vi "Simulated Acquisition Template (Host).vi"() -> ()   [LabVIEW 2016]
uses:
  <vilib>/FPGAPlugInAG/roboRIO/niLvFpga_Open_roboRIO.vi
  <vilib>/rvi/interface/common/dynamic/niFpgaDynamicAddResources.vi
  <vilib>/FPGAPlugInAG/Dynamic/niLvFpga_Download_Dynamic.vi
  <vilib>/FPGAPlugInAG/Dynamic/niLvFpga_Run_Dynamic.vi
  <vilib>/visionFPGA/Basics/Configure Image Transfer to Target/IMAQ FPGA Configure Image Transfer to Target U32.vi
  <vilib>/visionFPGA/Basics/Image Transfer to Target/IMAQ FPGA Image Transfer to Target U32.vi
  <vilib>/visionFPGA/Basics/Configure Image Transfer from Target/IMAQ FPGA Configure Image Transfer from Target U8.vi
  <vilib>/Utility/error.llb/Error Cluster From Error Code.vi
  <vilib>/rvi/errors/niLvFpgaAdjustHostInterfaceError.vi
  <vilib>/visionFPGA/Basics/Image Transfer from Target/IMAQ FPGA Image Transfer from Target U8.vi
  <vilib>/FPGAPlugInAG/Dynamic/niLvFpga_Close_Dynamic.vi
  <vilib>/rvi/interface/nirviOpenFPGA/nirviOpenFPGA.xnode
  FPGA Bitfiles/ImageProcessingw_FPGATarget2_ImageProcessingw_ZcF2hsHpmf8.lvbitx
  Image Processing with Vision Assistant (FPGA).vi
  <vilib>/rvi/interface/nirviMethod/nirviMethod.xnode
  <vilib>/rvi/interface/nirviReadWriteControl/nirviReadWriteControl.xnode
  <vilib>/rvi/interface/nirviCloseFPGA/nirviCloseFPGA.xnode
  <vilib>/visionFPGA/NI_VDM_FPGA_Basics.lvlib
  NiFpgaLv.dll
  <vilib>/rvi/interface/Simulation/niFpgaSimulationCallBeginRW.vi
panel:
  out "Image 2":T1(plugin-control)
  in  "Image Folder":path=path "/VISION/Images"
  out "Error Out":errorcluster
  out "Image":T1(plugin-control)
  in  "Stop":bool
  # "Overview: Demonstrates how to cycle through a folder of images, transfer the images to a FPGA target for processing, and retrieve the processed images for display or further processing on the host.\nRequirements:\n- LabVIEW FPGA\n- Vision Development Module\nInstructions:\n1. Select the folder containing the images to use.  For a Real-Time target it may be necessary to copy the images to the target first.\n2. Run the VI."
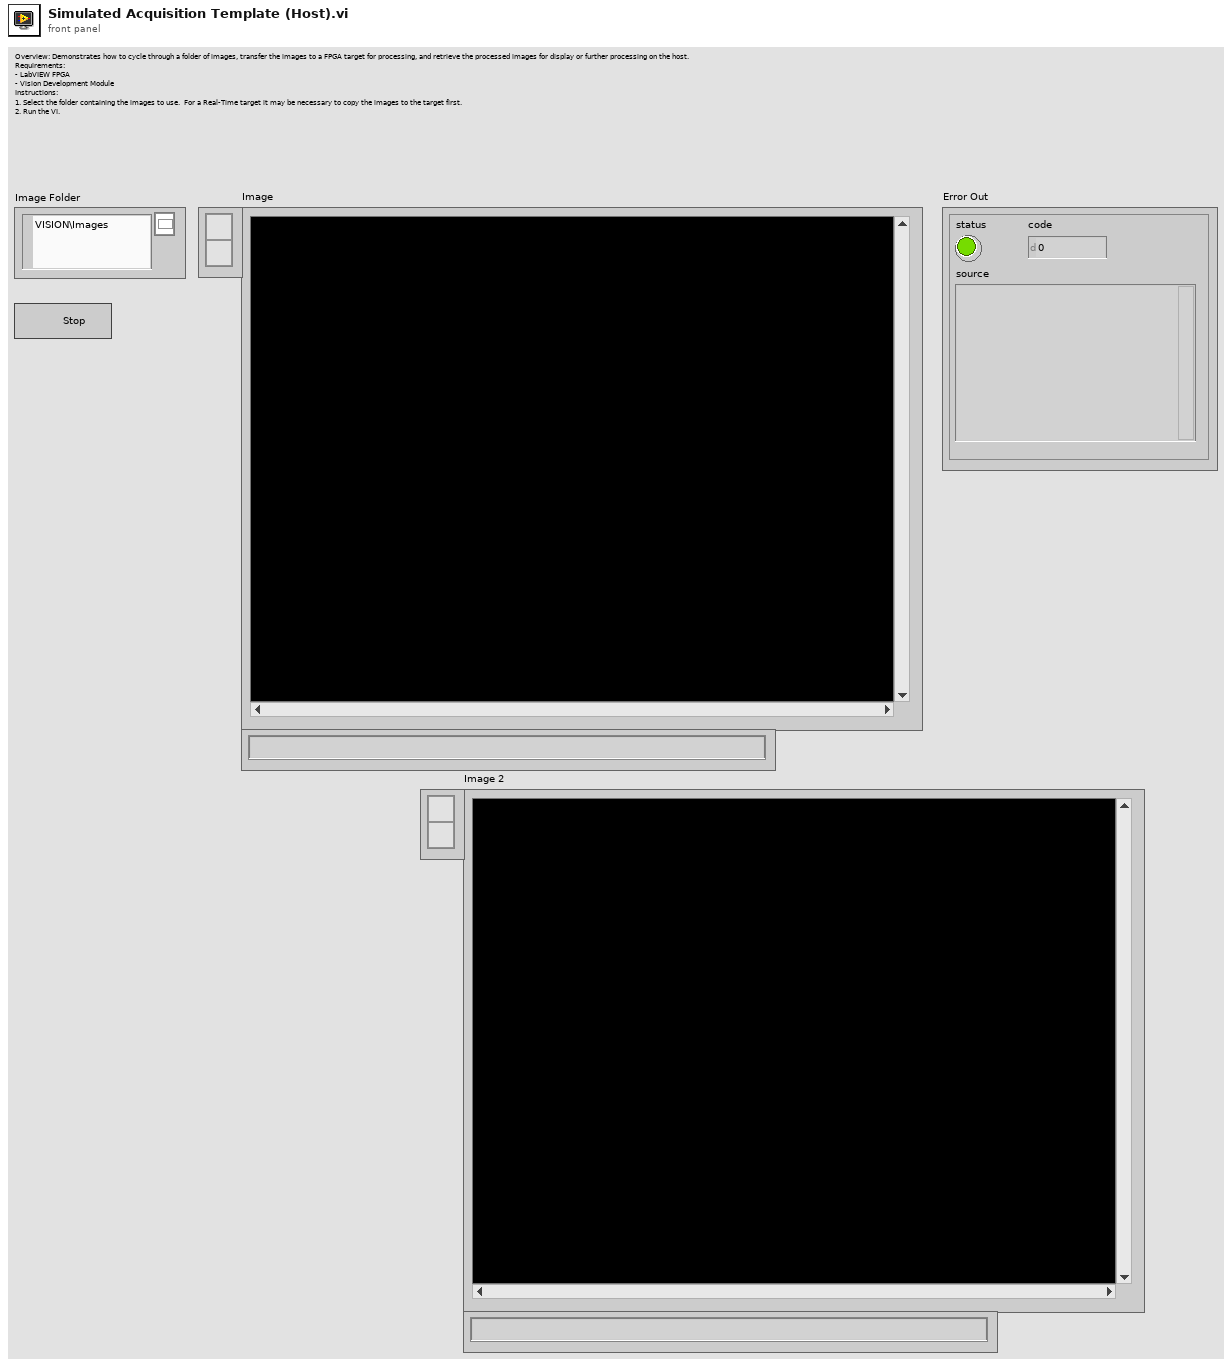
[diagram p1: front panel]
types:
  T1 = typedef "IMAQ Image.ctl" = refnum<image>
  T2 = typedef "Image Type" = u32
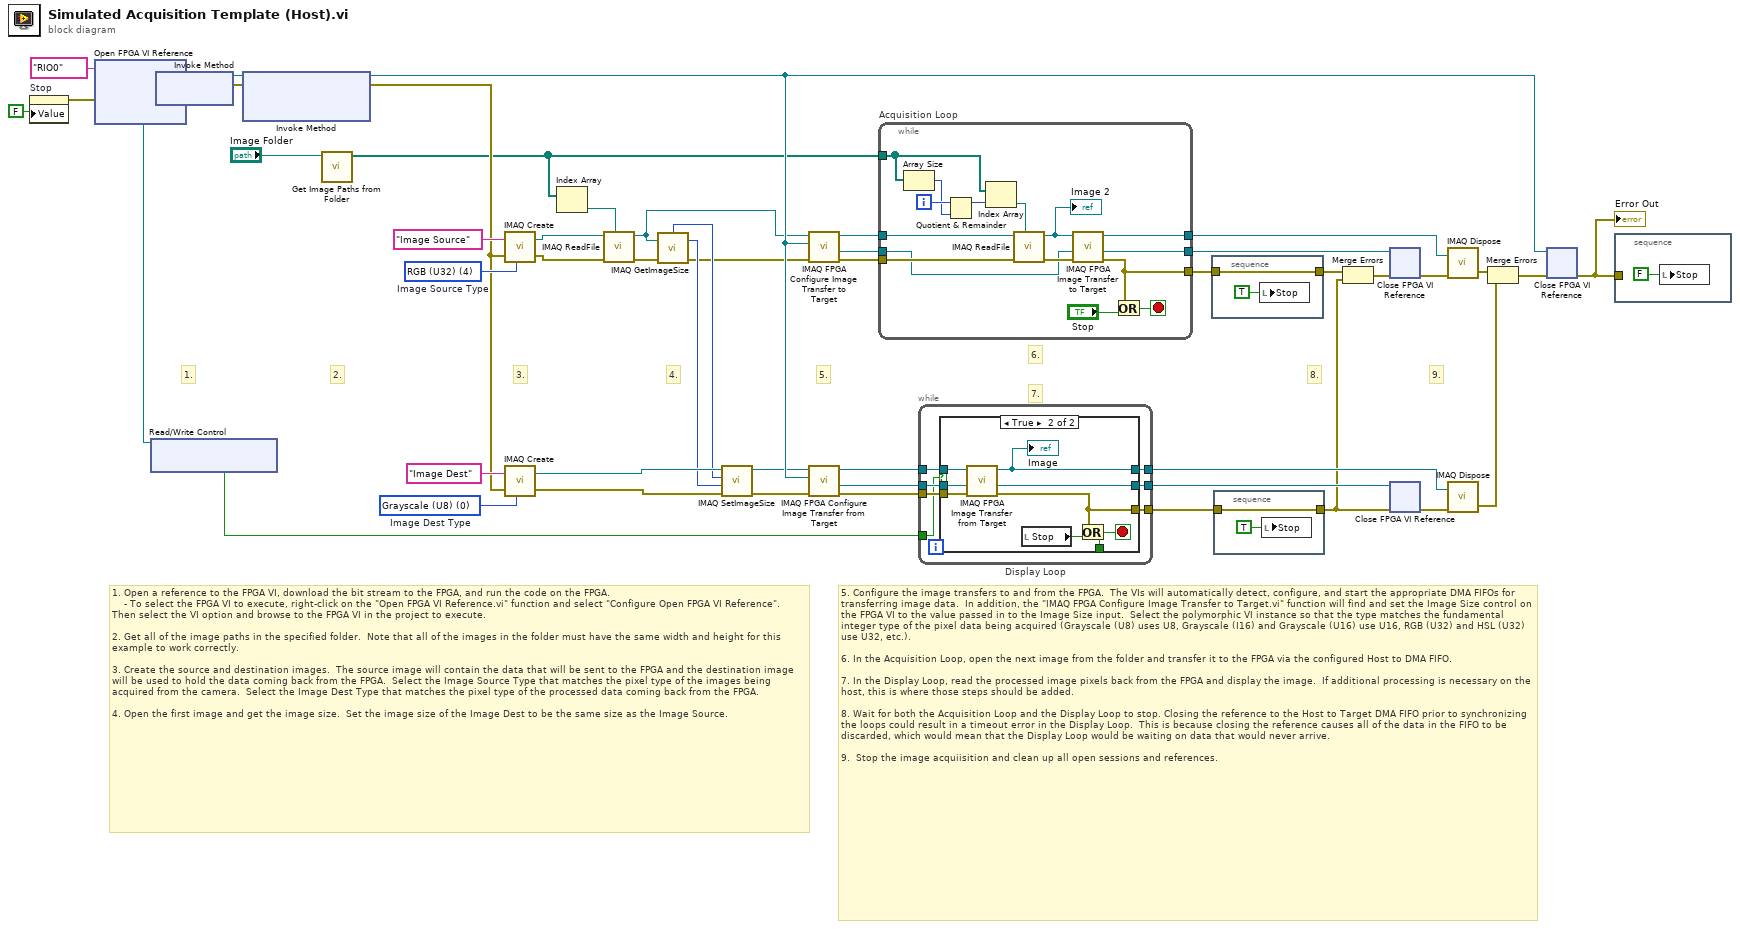
[diagram p0: block diagram]
diagram:
  w26 = T2 0 items=["Grayscale (U8)", "Grayscale (I16)", "Grayscale (SGL)", "Complex (CSG)", "RGB (U32)", "HSL (U32)", "RGB (U64)", "Grayscale (U16)"]  # Image Dest Type
  w27 = T2 4 items=["Grayscale (U8)", "Grayscale (I16)", "Grayscale (SGL)", "Complex (CSG)", "RGB (U32)", "HSL (U32)", "RGB (U64)", "Grayscale (U16)"]  # Image Source Type
  # "5. Configure the image transfers to and from the FPGA.  The VIs will automatically detect, configure, and start the appropriate DMA FIFOs for transferring image data.  In addition, the \"IMAQ FPGA Configure Image Transfer to Target.vi\" function will find and set the Image Size control on the FPGA VI to the value passed in to the Image Size input.  Select the polymorphic VI instance so that the type matches the fundamental integer type of the pixel data being acquired (Grayscale (U8) uses U8, Grayscale (I16) and Grayscale (U16) use U16, RGB (U32) and HSL (U32) use U32, etc.).\n\n6. In the Acquisition Loop, open the next image from the folder and transfer it to the FPGA via the configured Host to DMA FIFO.\n\n7. In the Display Loop, read the processed image pixels back from the FPGA and display the image.  If additional processing is necessary on the host, this is where those steps should be added.\n\n8. Wait for both the Acquisition Loop and the Display Loop to stop. Closing the reference to the Host to Target DMA FIFO prior to synchronizing the loops could result in a timeout error in the Display Loop.  This is because closing the reference causes all of the data in the FIFO to be discarded, which would mean that the Display Loop would be waiting on data that would never arrive.\n\n9.  Stop the image acquiisition and clean up all open sessions and references."
  # "1. Open a reference to the FPGA VI, download the bit stream to the FPGA, and run the code on the FPGA.\n    - To select the FPGA VI to execute, right-click on the \"Open FPGA VI Reference.vi\" function and select \"Configure Open FPGA VI Reference\".  Then select the VI option and browse to the FPGA VI in the project to execute.\n\n2. Get all of the image paths in the specified folder.  Note that all of the images in the folder must have the same width and height for this example to work correctly.\n\n3. Create the source and destination images.  The source image will contain the data that will be sent to the FPGA and the destination image will be used to hold the data coming back from the FPGA.  Select the Image Source Type that matches the pixel type of the images being acquired from the camera.  Select the Image Dest Type that matches the pixel type of the processed data coming back from the FPGA.\n\n4. Open the first image and get the image size.  Set the image size of the Image Dest to be the same size as the Image Source."
  # "9."
  # "8."
  # "7."
  # "6."
  # "5."
  # "4."
  # "3."
  # "2."
  # "1."
  n1 = property on="Stop" class="Bool (strict)"("Value"=FALSE ("Stop")) -> (error out=w46:errorcluster)  [unwired: 2 in, 1 out]
  n2 = xnode "Open FPGA VI Reference"("error in"=w46, "resource name"=tag "RIO0") -> ("FPGA VI Reference Out"=w2:refnum<k20>, "error out"=w43:errorcluster)
  n3 = xnode "Read/Write Control"("FPGA VI Reference In"=w2) -> ("ready to RecPic1 1"=w1:bool)  [unwired: 1 in, 2 out]
  n4 = xnode "Invoke Method"("FPGA VI Reference In"=w2, "error in"=w43) -> ("FPGA VI Reference Out"=w45:refnum<k20>, "error out"=w44:errorcluster)
  n5 = xnode "Invoke Method"("FPGA VI Reference In"=w45, "error in"=w44) -> ("FPGA VI Reference Out"=w28:refnum<k20>, "error out"=w10:errorcluster)  [unwired: 1 in]
  n6 = call "Get Image Paths from Folder.vi"("Image Folder"="Image Folder") -> ("Image Paths"=w7:path[])  [unwired: 10 in]
  n7 = call "IMAQ Create"("Image Name"="Image Source", "Image Type"=w27, "error in (no error)"=w10) -> ("New Image"=w19:T1, "error out"=w18:errorcluster)  [unwired: 2 in]
  n8 = call "IMAQ Create"("Image Name"="Image Dest", "Image Type"=w26, "error in (no error)"=w10) -> ("New Image"=w16:T1, "error out"=w14:errorcluster)  [unwired: 2 in]
  n9 = Index Array(array=w7) -> (element=w20:path)  [unwired: 1 in]
  n10 = call "IMAQ ReadFile"("File Path"=w20, "error in (no error)"=w18, "Image"=w19) -> ("error out"=w17:errorcluster, "Image Out"=w9:T1)  [unwired: 4 in, 3 out]
  n11 = call "IMAQ GetImageSize"("Image"=w9, "error in (no error)"=w17) -> ("Y Resolution"=w11:i32, "X Resolution"=w12:i32, "error out"=w8:errorcluster)  [unwired: 2 in]
  n12 = call "IMAQ SetImageSize"("error in (no error)"=w14, "Y Resolution"=w11, "X Resolution"=w12, "Image"=w16) -> ("error out"=w13:errorcluster, "Image Out"=w15:T1)  [unwired: 1 in]
  n13 = call-poly <vilib>:"IMAQ FPGA Configure Image Transfer to Target.vi"("error in (no error)"=w8, "FPGA VI Reference In"=w28, "Image"=w9) -> ("error out"=w4:errorcluster, "DMA FIFO Reference Out"=w5:refnum<k20>, "Image Out"=w6:T1)  [unwired: 5 in, 1 out]
  n14 = call-poly <vilib>:"IMAQ FPGA Configure Image Transfer from Target.vi"("error in (no error)"=w13, "FPGA VI Reference In"=w28, "Image"=w15) -> ("error out"=w41:errorcluster, "DMA FIFO Reference Out"=w40:refnum<k20>, "Image Out"=w42:T1)  [unwired: 6 in]
  n15 = while "Acquisition Loop" {
    tunnel: [w60] -> w24
    tunnel: w6 -> [w55]
    tunnel: w5 -> [w52]
    tunnel: [w62] -> w25
    tunnel: [w61] -> w39
    tunnel: w7 -> [w57]
    tunnel: w4 -> [w53]
    i -> [w59]
    stop <- w63 stop-if-true
    n16 = Array Size(array=w57) -> (size(s)=w58:i32)
    n17 = Quotient & Remainder(x=w59, y=w58) -> (x-y*floor(x/y)=w51:i32)  [unwired: 1 out]
    n18 = Index Array(array=w57, index=w51) -> (element=w54:path)
    n19 = call "IMAQ ReadFile"("File Path"=w54, "error in (no error)"=w53, "Image"=w55) -> ("error out"=w56:errorcluster, "Image Out"=w50:T1)  [unwired: 4 in, 3 out]
    "Image 2" <- w50
    n20 = call-poly <vilib>:"IMAQ FPGA Image Transfer to Target.vi"("error in (no error)"=w56, "DMA FIFO Reference In"=w52, "Image"=w50) -> ("error out"=w60:errorcluster, "DMA FIFO Reference Out"=w62:refnum<k20>, "Image Out"=w61:T1)  [unwired: 6 in]
    n21 = Or(x=w60, y="Stop") -> (x .or. y?=w63:bool)
  }
  n22 = while "Display Loop" {
    tunnel: w42 -> [w71]
    tunnel: [w70] -> w36
    tunnel: w41 -> [w69]
    tunnel: w40 -> [w68]
    tunnel: [w67] -> w37
    tunnel: [w66] -> w34
    tunnel: w1 -> [w65]
    stop <- w72 stop-if-true
    n23 = case shown="True" w65 {
      tunnel: [_ w83] -> w72
      tunnel: w71 -> [w75 w82]
      tunnel: [w75 w81] -> w70
      tunnel: w69 -> [w73 w80]
      tunnel: w68 -> [w74 w79]
      tunnel: [w74 w78] -> w67
      tunnel: [w73 w77] -> w66
      frame False {
      }
      frame True {
        n24 = call-poly <vilib>:"IMAQ FPGA Image Transfer from Target.vi"("error in (no error)"=w80, "DMA FIFO Reference In"=w79, "Image"=w82) -> ("error out"=w77:errorcluster, "DMA FIFO Reference Out"=w78:refnum<k20>, "Image Out"=w81:T1)  [unwired: 6 in]
        "Image" <- w81
        n25 = local read "Stop"() -> (w76:bool)
        n26 = Or(x=w77, y=w76) -> (x .or. y?=w83:bool)
      }
    }
  }
  n27 = stacked-sequence {
    tunnel: w24 -> [w84]
    tunnel: [w84] -> w22
    frame #0 {
      n28 = local write "Stop"(TRUE ("Stop")) -> ()
    }
  }
  n29 = stacked-sequence {
    tunnel: w34 -> [w86]
    tunnel: [w86] -> w23
    frame #0 {
      n30 = local write "Stop"(TRUE ("Stop")) -> ()
    }
  }
  n31 = Merge Errors(w22, w23) -> (w21:errorcluster)
  n32 = xnode "Close FPGA VI Reference"("FPGA VI Reference In"=w25, "error in"=w21) -> ("error out"=w38:errorcluster)
  n33 = xnode "Close FPGA VI Reference"("FPGA VI Reference In"=w37, "error in"=w23) -> ("error out"=w35:errorcluster)
  n34 = call "IMAQ Dispose"("Image"=w39, "error in (no error)"=w38) -> ("error out"=w32:errorcluster)  [unwired: 4 in]
  n35 = call "IMAQ Dispose"("Image"=w36, "error in (no error)"=w35) -> ("error out"=w33:errorcluster)  [unwired: 4 in]
  n36 = Merge Errors(w32, w33) -> (w30:errorcluster)
  n37 = xnode "Close FPGA VI Reference"("FPGA VI Reference In"=w28, "error in"=w30) -> ("error out"=w29:errorcluster)
  "Error Out" <- w29
  n38 = stacked-sequence {
    tunnel: w29 -> [_]
    frame #0 {
      n39 = local write "Stop"(FALSE ("Stop")) -> ()
    }
  }
